vi "MC_Get_Selections.vi"(8 "error in (no error)":errorcluster, 11 "MCin":refnum<vi>) -> (0 "error out":errorcluster, 1 "TestRows":i32[](array[numeric]), 2 "TestNames":string[](array[string]), 3 "MCout":refnum<vi>, 5 "TestItems":string[][](array[string]))   [LabVIEW 2013]
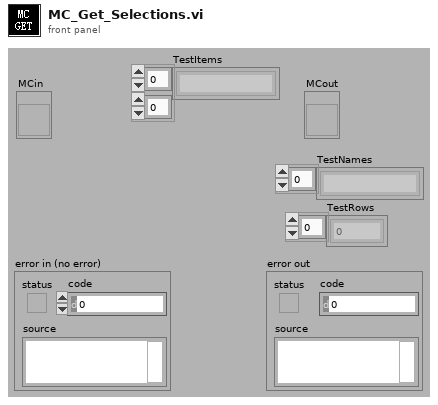
[diagram p1: front panel]
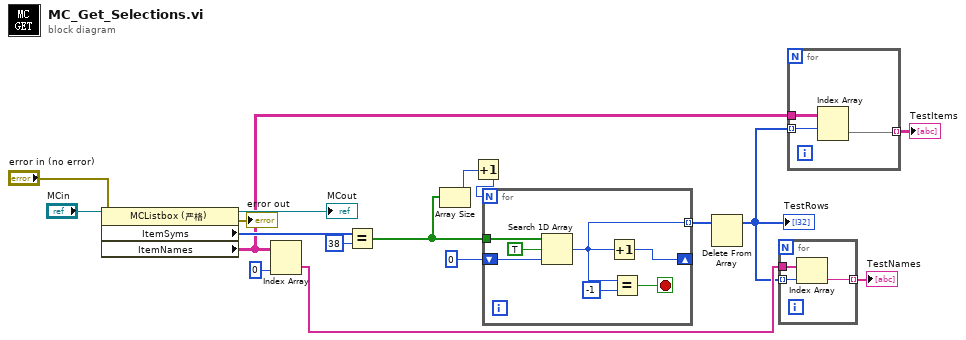
[diagram p0: block diagram]
diagram:
  n1 = property on="属性节点" class="MCListbox (严格)"(reference="MCin", error in="error in (no error)") -> (reference out=→"MCout":refnum<vi>, error out=→"error out":errorcluster, "ItemSyms"=w15:i32[], "ItemNames"=w6:string[][])
  n2 = Index Array(array=w6, index (col)=0 ("禁用的索引 (列)")) -> (element=w10:string[])  [unwired: 1 in]
  n3 = Equal?(x=w15, y=38) -> (x = y?=w8:bool[])
  n4 = Array Size(array=w8) -> (size(s)=w3:i32)
  n5 = Increment(x=w3) -> (x+1=w4:i32)
  n6 = for {
    N: w4 -> [_]
    tunnel: w8 -> [w24]
    shift-right: [w22] -> _
    shift-left: 0 -> [w21]
    tunnel: [w18] -> w11 mode=indexing
    stop <- w20 stop-if-true
    n7 = Search 1D Array(1D array=w24, element=TRUE ("元素"), start index (0)=w21) -> (index of element=w18:i32)
    n8 = Increment(x=w18) -> (x+1=w22:i32)
    n9 = Equal?(x=w18, y=-1) -> (x = y?=w20:bool)
  }
  n10 = Delete From Array(array=w11) -> (array with subset deleted=w7:i32[])  [unwired: 2 in, 1 out]
  "TestRows" <- w7
  n11 = for {
    tunnel: w10 -> [w27]
    tunnel: w7 -> [w26] mode=indexing
    tunnel: [w25] -> w9 mode=indexing
    n12 = Index Array(array=w27, index=w26) -> (element=w25:string)
  }
  "TestNames" <- w9
  n13 = for {
    tunnel: w7 -> [w29] mode=indexing
    tunnel: w6 -> [w30]
    tunnel: [w28] -> w5 mode=indexing
    n14 = Index Array(array=w30, index (row)=w29) -> (element=w28:string[])  [unwired: 1 in]
  }
  "TestItems" <- w5
